vi "ExecuteMultipleFilesProcessing.vi"(8 "Callback queue in":refnum<queue>, 9 "Path":refnum<vi>, 10 "CalcPeakAreas":refnum<vi>, 11 "Accumulate":refnum<vi>) -> ()   [LabVIEW 2012]
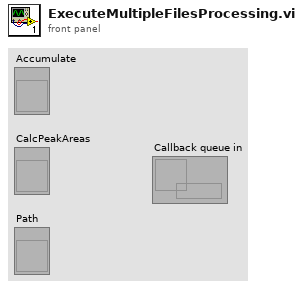
[diagram p1: front panel]
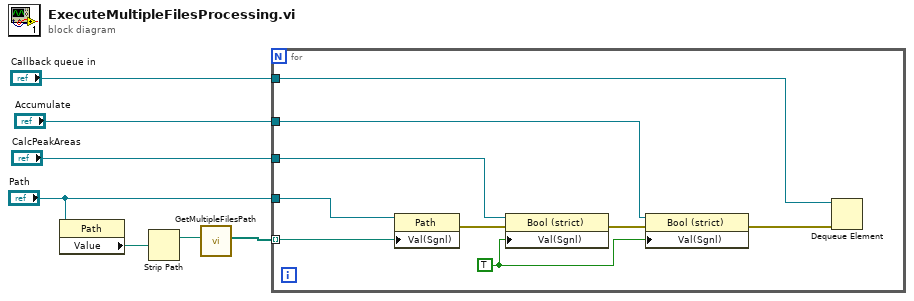
[diagram p0: block diagram]
diagram:
  n1 = property class="Path"(reference="Path") -> ("Value"=w3:path)  [unwired: 1 in, 2 out]
  n2 = Strip Path(path=w3) -> (stripped path=w4:path)  [unwired: 1 out]
  n3 = call "GetMultipleFilesPath.vi"("Path"=w4) -> ("PathArray"=w2:path[])  [unwired: 10 in]
  n4 = for {
    tunnel: w2 -> [w13] mode=indexing
    tunnel: "Path" -> [w12]
    tunnel: "CalcPeakAreas" -> [w11]
    tunnel: "Accumulate" -> [w10]
    tunnel: "Callback queue in" -> [w9]
    w16 = TRUE
    n5 = property class="Path"(reference=w12, "Val(Sgnl)"=w13) -> (error out=w14:errorcluster)  [unwired: 1 in, 1 out]
    n6 = property class="Bool (strict)"(reference=w11, error in=w14, "Val(Sgnl)"=w16) -> (error out=w15:errorcluster)  [unwired: 1 out]
    n7 = property class="Bool (strict)"(reference=w10, error in=w15, "Val(Sgnl)"=w16) -> (error out=w8:errorcluster)  [unwired: 1 out]
    n8 = Dequeue Element(queue=w9, error in (no error)=w8) -> ()  [unwired: 1 in, 4 out]
  }
